vi "Get Foreign Key.vi"(8 "error in (no error)":errorcluster, 9 "Column Name Array (All Columns)":string[](array[string]), 10 "Table Name":string, 11 "ADODB in":refnum<class "ADODB.lvclass">) -> (0 "error out":errorcluster, 2 "FK Properties Array":T1[](array[typedef]), 3 "ADODB out":refnum<class "ADODB.lvclass">)   [LabVIEW 2020, in "ADODB.lvlib" / "ADODB.lvclass"]
uses:
  ADODB.lvclass
  Database/foreign key properties.ctl
  ADODB.lvclass/ADODB.ctl
  <vilib>/addons/database/NI_Database_API.lvlib
  ADODB.lvlib
  Database Interfaces.lvlib
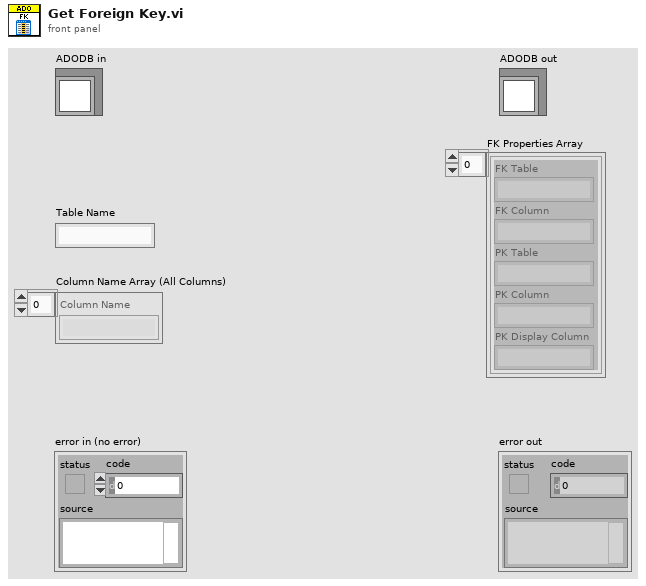
[diagram p1: front panel]
types:
  T1 = typedef "Database Interfaces.lvlib/foreign key properties.ctl" = cluster{"FK Table":string, "FK Column":string, "PK Table":string, "PK Column":string, "PK Display Column":string}
  T2 = cluster{"Parent Table":string, "Parent Column":string, "Foreign Table":string, "Foreign PK Column":string, "Foreign Display Column":string}[]
  T3 = typedef "NI_Database_API.lvlib/Conn ObjectReference.ctl" = refnum<k1>
  T4 = typedef "NI_Database_API.lvlib/Conn DataMembers.ctl" = cluster{"ADODB._Connection":refnum<k7>, "recordset objects":i32, "command objects":i32}
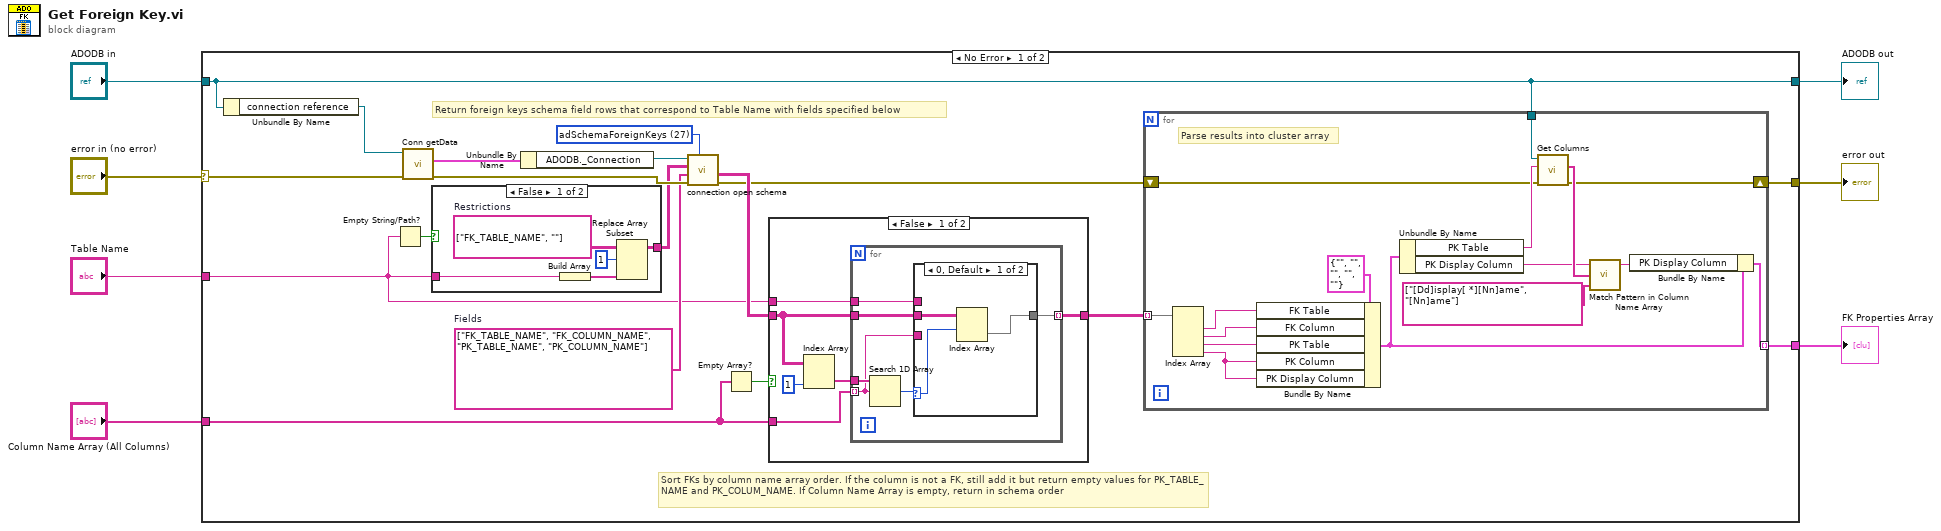
[diagram p0: block diagram]
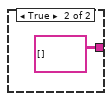
[diagram p2: hidden frame]
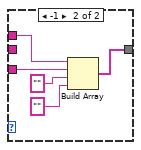
[diagram p3: hidden frame]
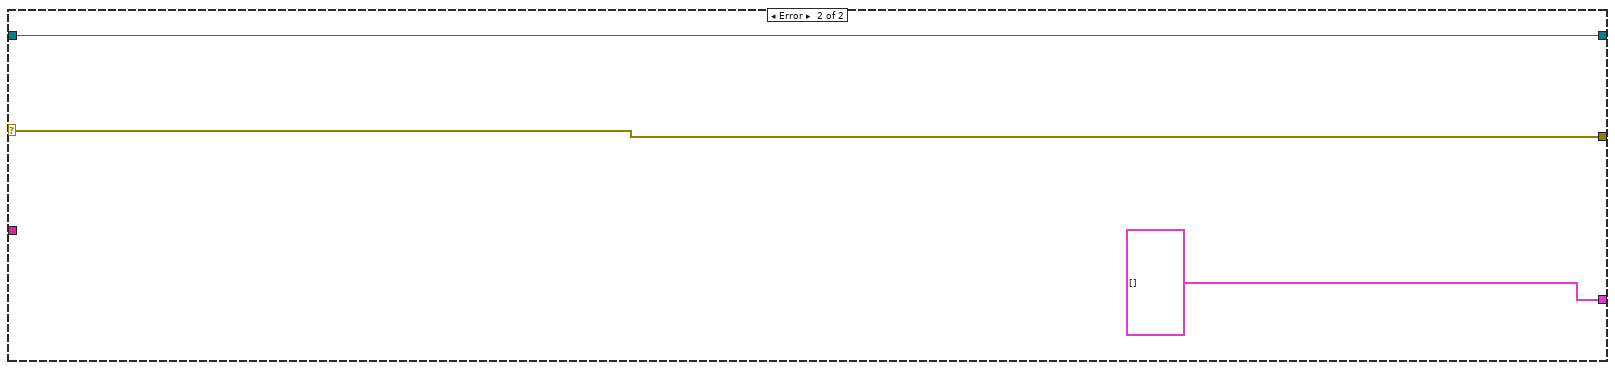
[diagram p5: hidden frame]
diagram:
  n1 = case shown="No Error" "error in (no error)" {
    selector: "error in (no error)" -> [w11 w71]
    tunnel: "ADODB in" -> [w10 w70]
    tunnel: [w10 w70] -> w6
    tunnel: [w23 T2 []] -> w1
    tunnel: "Table Name" -> [w14 _]
    tunnel: "Column Name Array (All Columns)" -> [w17 _]
    tunnel: [w8 w71] -> w2
    frame No Error {
      w20 = string[] ["FK_TABLE_NAME", "FK_COLUMN_NAME", "PK_TABLE_NAME", "PK_COLUMN_NAME"]  # Fields
      w21 = 27 items=["adSchemaProviderSpecific"=-1, "adSchemaAsserts"=0, "adSchemaCatalogs"=1, "adSchemaCharacterSets"=2, "adSchemaCollations"=3, "adSchemaColumns"=4, "adSchemaCheckConstraints"=5, "adSchemaConstraintColumnUsage"=6, "adSchemaConstraintTableUsage"=7, "adSchemaKeyColumnUsage"=8, "adSchemaReferentialContraints, adSchemaReferentialConstraints"=9, "adSchemaTableConstraints"=10, "adSchemaColumnsDomainUsage"=11, "adSchemaIndexes"=12, "adSchemaColumnPrivileges"=13, "adSchemaTablePrivileges"=14, "adSchemaUsagePrivileges"=15, "adSchemaProcedures"=16, "adSchemaSchemata"=17, "adSchemaSQLLanguages"=18, "adSchemaStatistics"=19, "adSchemaTables"=20, "adSchemaTranslations"=21, "adSchemaProviderTypes"=22, "adSchemaViews"=23, "adSchemaViewColumnUsage"=24, "adSchemaViewTableUsage"=25, "adSchemaProcedureParameters"=26, "adSchemaForeignKeys"=27, "adSchemaPrimaryKeys"=28, "adSchemaProcedureColumns"=29, "adSchemaDBInfoKeywords"=30, "adSchemaDBInfoLiterals"=31, "adSchemaCubes"=32, "adSchemaDimensions"=33, "adSchemaHierarchies"=34, "adSchemaLevels"=35, "adSchemaMeasures"=36, "adSchemaProperties"=37, "adSchemaMembers"=38, "adSchemaTrustees"=39] ("Schema")
      # "Return foreign keys schema field rows that correspond to Table Name with fields specified below"
      # "Sort FKs by column name array order. If the column is not a FK, still add it but return empty values for PK_TABLE_NAME and PK_COLUM_NAME. If Column Name Array is empty, return in schema order"
      n2 = Unbundle By Name(w10) -> ("connection reference"=w12:T3)
      n3 = Empty String/Path?(string/path=w14) -> (empty?=w13:bool)
      n4 = call <vilib>:"Conn getData.vi"("error in (no error)"=w11, "connection reference"=w12) -> ("error out"=w22:errorcluster, "data"=w24:T4)  [unwired: 2 in, 2 out]
      n5 = case shown="False" w13 {
        tunnel: [w27 string[][] [] ("Restrictions")] -> w19
        tunnel: w14 -> [w26 _]
        frame False {
          w30 = string[][] [["FK_TABLE_NAME"], [""]]  # Restrictions
          n6 = Build Array(w26) -> (w28:string[])
          n7 = Replace Array Subset(array=w30, new element=w28, index (row)=1) -> (w27:string[][])  [unwired: 1 in]
        }
        frame True {
        }
      }
      n8 = Unbundle By Name(w24) -> ("ADODB._Connection"=w25:refnum<k7>)
      n9 = call "connection open schema.vi"("Schema"=w21, "error in (no error)"=w22, "Fields"=w20, "Restrictions"=w19, "ADODB._Connection"=w25) -> ("error out"=w9:errorcluster, "Schema Out"=w16:string[][])  [unwired: 3 in, 2 out]
      n10 = Empty Array?(array=w17) -> (empty?=w18:bool)
      n11 = case shown="False" w18 {
        tunnel: w16 -> [w36 w52]
        tunnel: w17 -> [w37 _]
        tunnel: [w32 w52] -> w15
        tunnel: w14 -> [w33 _]
        frame False {
          n12 = Index Array(array=w36, index (col)=1 ("disabled index (col)")) -> (element=w35:string[])  [unwired: 1 in]
          n13 = for {
            tunnel: w37 -> [w39] mode=indexing
            tunnel: w36 -> [w41]
            tunnel: w35 -> [w43]
            tunnel: w33 -> [w40]
            tunnel: [w38] -> w32 mode=indexing
            n14 = Search 1D Array(1D array=w43, element=w39) -> (index of element=w42:i32)  [unwired: 1 in]
            n15 = case shown="0, Default" w42 {
              selector: w42 -> [w45 _]
              tunnel: w41 -> [w46 _]
              tunnel: w40 -> [_ w51]
              tunnel: w39 -> [_ w48]
              tunnel: [w44 w47] -> w38
              frame 0, Default {
                n16 = Index Array(array=w46, index (row)=w45) -> (element=w44:string[])  [unwired: 1 in]
              }
              frame -1 {
                n17 = Build Array(w51, w48, "" ("element"), "" ("element")) -> (w47:string[])
              }
            }
          }
        }
        frame True {
        }
      }
      n18 = for {
        tunnel: [w54] -> w23 mode=indexing
        tunnel: w15 -> [w68] mode=indexing
        tunnel: w10 -> [w62]
        shift-right: [w56] -> w8
        shift-left: w9 -> [w57]
        # "Parse results into cluster array"
        n19 = Index Array(array=w68) -> (element #1=w67:string, element #2=w66:string, element #3=w65:string, element #4=w64:string)  [unwired: 4 in]
        n20 = Bundle By Name(cluster=T1 {"FK Table"="", "FK Column"="", "PK Table"="", "PK Column"="", "PK Display Column"=""} ("Foreign Key"), "FK Table"=w67, "FK Column"=w66, "PK Table"=w65, "PK Column"=w64, "PK Display Column"=w64) -> (w55:T1)
        n21 = Unbundle By Name(w55) -> ("PK Table"=w61:string, "PK Display Column"=w59:string)
        n22 = call-dynamic "Get Columns.vi"("error in (no error)"=w57, "Table Name"=w61, "ADODB in"=w62) -> ("error out"=w56:errorcluster, "Column Name Array"=w60:string[])  [unwired: 6 in, 1 out]
        n23 = call "Match Pattern in Column Name Array.vi"("Match Pattern Regex"=string[] ["[Dd]isplay[ *][Nn]ame", "[Nn]ame"], "Column Name Array"=w60, "Not Found Name"=w59) -> ("Matching Name"=w53:string)  [unwired: 2 out]
        n24 = Bundle By Name(cluster=w55, "PK Display Column"=w53) -> (w54:T1)
      }
    }
    frame Error {
    }
  }
  "error out" <- w2
  "ADODB out" <- w6
  "FK Properties Array" <- w1
